vi "test_sendmail.vi"() -> ()   [LabVIEW 2019]
panel:
  in  "message":string="TEST." caption="Message"
  in  "title":string="test_sendmail.vi"
  in  "address_array":string[](array[string])
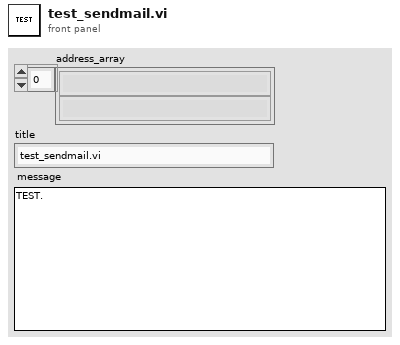
[diagram p1: front panel]
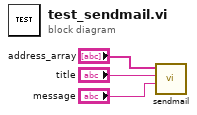
[diagram p0: block diagram]
diagram:
  n1 = call "sendmail.vi"("message"="message", "title"="title", "address_array"="address_array") -> ()  [unwired: 8 in, 1 out]
